vi "LEP_RV_MsgBox2Buttons.vi"(8 "Message":string, 9 "Button 2 Text":string="Cancel", 10 "Button 1 Text":string="OK", 11 "µVision":string="µVision") -> (3 "Button 1 Pressed":bool)   [LabVIEW 2011]
doc: "Displays <B>Error Message</B> and <B>Error Output</B> in the <B>Failed to build executable</B> dialog box."
panel:
  out "Text":string
  in  "Button 1":bool
  in  "Button 2":bool
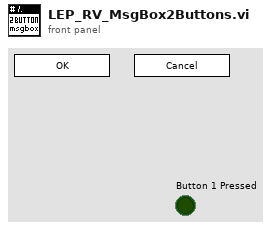
[diagram p1: front panel]
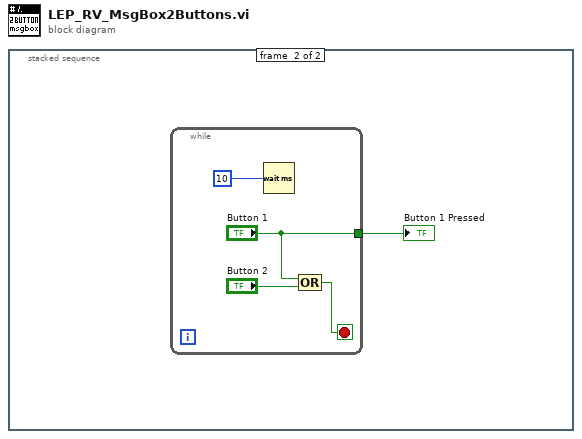
[diagram p0: block diagram]
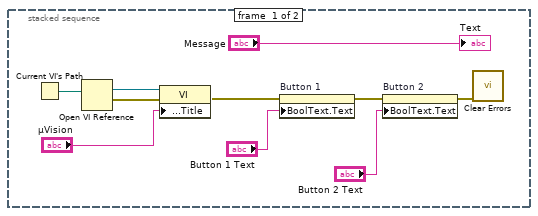
[diagram p2: hidden frame]
diagram:
  n1 = stacked-sequence {
    frame #0 {
      n2 = Current VI's Path() -> (path=w10:path)
      n3 = Open VI Reference(vi path=w10) -> (vi reference=w9:refnum<vi>, error out=w8:errorcluster)  [unwired: 1 in, 4 out]
      n4 = property class="VI"(reference=w9, error in=w8, "Front Panel.Title"="µVision") -> (error out=w3:errorcluster)  [unwired: 1 out]
      n5 = property on="Button 1" class="Bool"(error in=w3, "BoolText.Text"="Button 1 Text") -> (error out=w2:errorcluster)  [unwired: 1 in, 1 out]
      n6 = property on="Button 2" class="Bool"(error in=w2, "BoolText.Text"="Button 2 Text") -> (error out=w6:errorcluster)  [unwired: 1 in, 1 out]
      n7 = call <vilib>:"Clear Errors.vi"("error in (no error)"=w6) -> ()  [unwired: 7 out]
      "Text" <- "Message"
    }
    frame #1 {
      n8 = while {
        tunnel: ["Button 1"] -> w11
        stop <- w14 stop-if-true
        n9 = Wait (ms)(milliseconds to wait=u32 10) -> ()  [unwired: 1 out]
        n10 = Compound Arithmetic op=OR("Button 1", "Button 2") -> (w14:bool)
      }
      "Button 1 Pressed" <- w11
    }
  }
